vi "S2C_Shared_Proc_ErrorEvent.vi"(8 "Error In":errorcluster, 11 "Command":string) -> (0 "Error Out":errorcluster)   [LabVIEW 2024]
doc: "Performs a lookup of the custom error code and appends any additional information to the error."
uses:
  <vilib>/Utility/error.llb/DialogType.ctl
  <vilib>/Utility/error.llb/Trim Whitespace One-Sided.vi
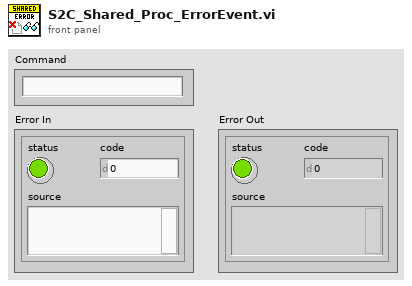
[diagram p1: front panel]
types:
  T1 = typedef "DialogType.ctl" = u16
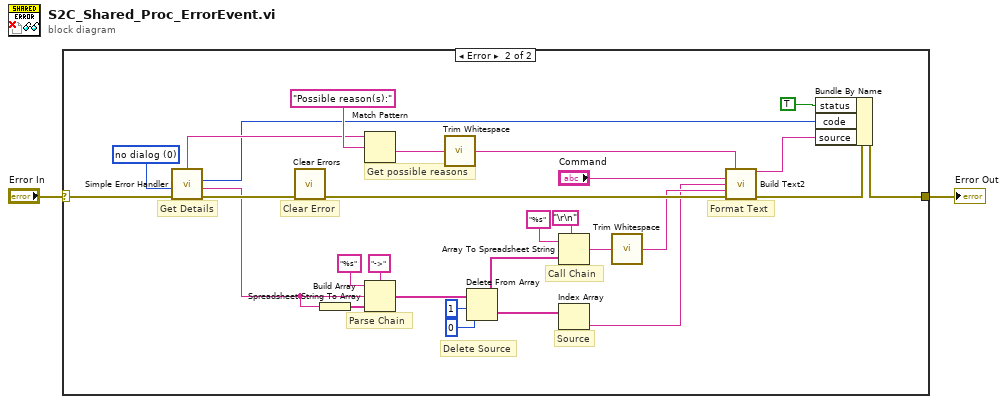
[diagram p0: block diagram]
diagram:
  n1 = case shown="Error" "Error In" {
    selector: "Error In" -> [w3 w8]
    tunnel: [w3 w10] -> w2
    frame No Error {
    }
    frame Error {
      w9 = T1 0 items=["no dialog", "OK message", "continue or stop message", "OK message + warnings", "continue/stop + warnings"] ("type of dialog (OK msg:1)")
      # "Get Details"
      # "Clear Error"
      # "Get possible reasons"
      # "Parse Chain"
      # "Delete Source"
      # "Source"
      # "Call Chain"
      # "Format Text"
      n2 = call <vilib>:"Simple Error Handler.vi"("type of dialog (OK msg:1)"=w9, "error in (no error)"=w8) -> ("code out"=w4:i32, "source out"=w6:string, "error out"=w7:errorcluster, "message"=w5:string)  [unwired: 3 in, 1 out]
      n3 = call <vilib>:"Clear Errors.vi"("error in (no error)"=w7) -> ("error out"=w18:errorcluster)  [unwired: 5 in, 1 out]
      n4 = Build Array(w6) -> (w30:string[])
      n5 = Match Pattern(string=w5, regular expression="Possible reason(s):") -> (after substring=w19:string)  [unwired: 1 in, 3 out]
      n6 = Spreadsheet String To Array(delimiter (Tab)="->", format string="%s", spreadsheet string=w6, array type (2D Dbl)=w30) -> (array=w28:string[])
      n7 = call <vilib>:"Trim Whitespace.vi"("string"=w19) -> ("trimmed string"=w12:string)  [unwired: 1 in]
      n8 = Delete From Array(array=w28, length=1, index=0) -> (deleted portion=w25:string[], array with subset deleted=w24:string[])
      n9 = Array To Spreadsheet String(delimiter (Tab)="\r\n", array=w24, 3:"%s" ("format string")) -> (spreadsheet string=w21:string)
      n10 = Index Array(array=w25) -> (element=w11:string)  [unwired: 1 in]
      n11 = call <vilib>:"Trim Whitespace.vi"("string"=w21) -> ("trimmed string"=w14:string)  [unwired: 1 in]
      n12 = call "Build Text2"("Reason"=w12, "Cmd"="Command", "Source"=w11, "Chain"=w14, "error in (no error)"=w18) -> ("Result"=w16:string, "error out"=w17:errorcluster)  [unwired: 9 in]
      n13 = Bundle By Name(cluster=w17, "status"=TRUE, "code"=w4, "source"=w16) -> (w10:errorcluster)
    }
  }
  "Error Out" <- w2
